vi "Write_DataLog.vi"   [LabVIEW 2018]
types:
  T1 = enum16{"open", "replace", "create", "open or create", "replace or create", "replace or create with confirmation"}
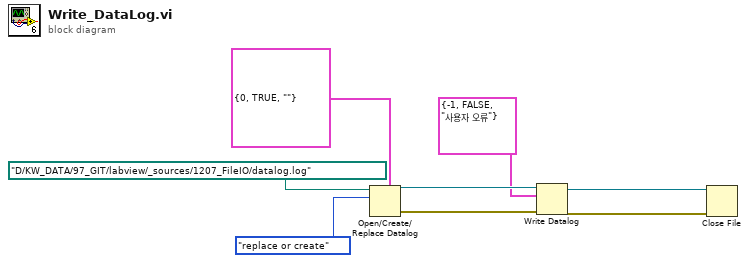
[diagram p0: block diagram]
diagram:
  n1 = Open/Create/Replace Datalog(5:cluster{i32, bool, string} {0, TRUE, ""}, 10:T1."replace or create" ("동작(0:open)"), 11:path "D:/KW_DATA/97_GIT/labview/_sources/1207_FileIO/datalog.log" ("데이터로그 경로(대화 상자 사용)")) -> (0:w6:errorcluster, 3:w7:refnum<k1>)  [unwired: 3 in, 1 out]
  n2 = Write Datalog(4:w6, 6:cluster{i32, bool, string} {-1, FALSE, "사용자 오류"} ("레코드"), 7:w7) -> (0:w4:errorcluster, 3:w5:refnum<k1>)
  n3 = Close File(refnum=w5, error in=w4) -> ()  [unwired: 2 out]
